vi "Test Performance.vi"() -> ()   [LabVIEW 2019]
uses:
  src/Typedefs/Interpolation Configuration--cluster.ctl
  <vilib>/Analysis/baseanly.llb/Mean.vi
  <vilib>/Analysis/baseanly.llb/Mean (DBL).vi
  src/xy_utilities.lvlib
panel:
  in  "Configure":T1={"X Low"=0.0, "X High"=1.0, "X Step"=0.1, "Fake Point"=0.0} {"Fake Point" format="%#_6p"; "X Step" format="%#_6p"; "X High" format="%#_6p"; "X Low" format="%#_6p"}
  out "XY Data 3":cluster{"X-array":dbl[], dbl[]}[](graph)
  out "Intensity Graph 2":dbl[][](graph)
  out "Intensity Graph":dbl[][](graph)
  out "execution time (s)":dbl
  out "XY Data 2":cluster{"X-array":dbl[], "Y-array":dbl[]}(graph)
  out "XY Data":cluster{"X-array":dbl[], "Y-array":dbl[]}(graph)
  # "0: 21\"\n5: 0.09\""
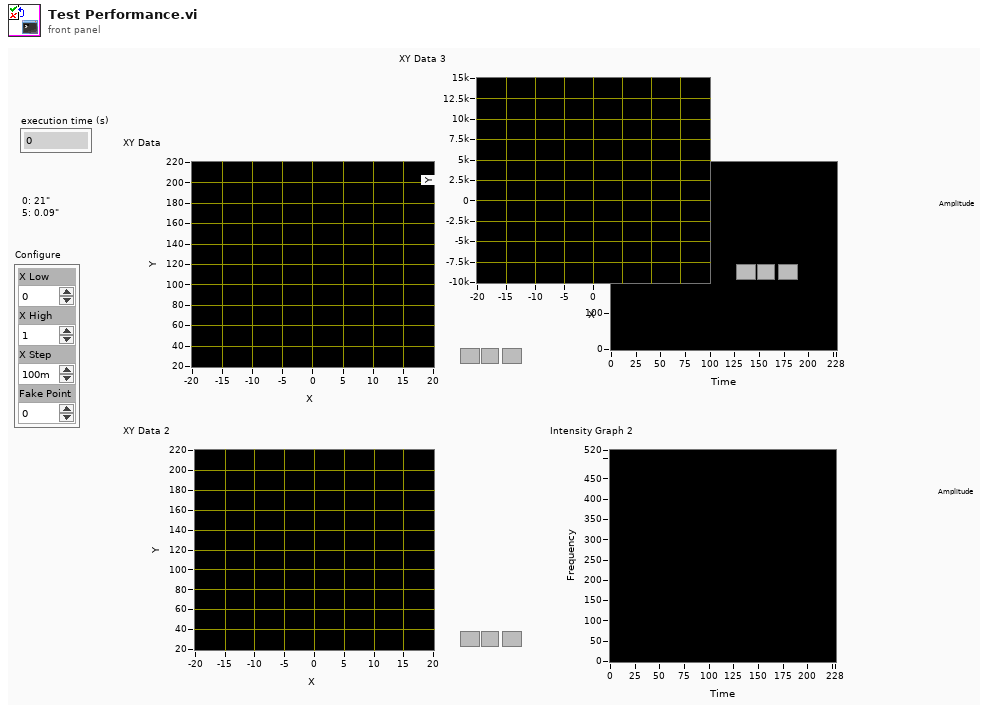
[diagram p1: front panel]
types:
  T1 = typedef "xy_utilities.lvlib/Interpolation Configuration--cluster.ctl" = cluster{"X Low":dbl, "X High":dbl, "X Step":dbl, "Fake Point":dbl}
  T2 = enum16{"thermal waveguide", "superlattice waveguide", "decay in atmosphere"}
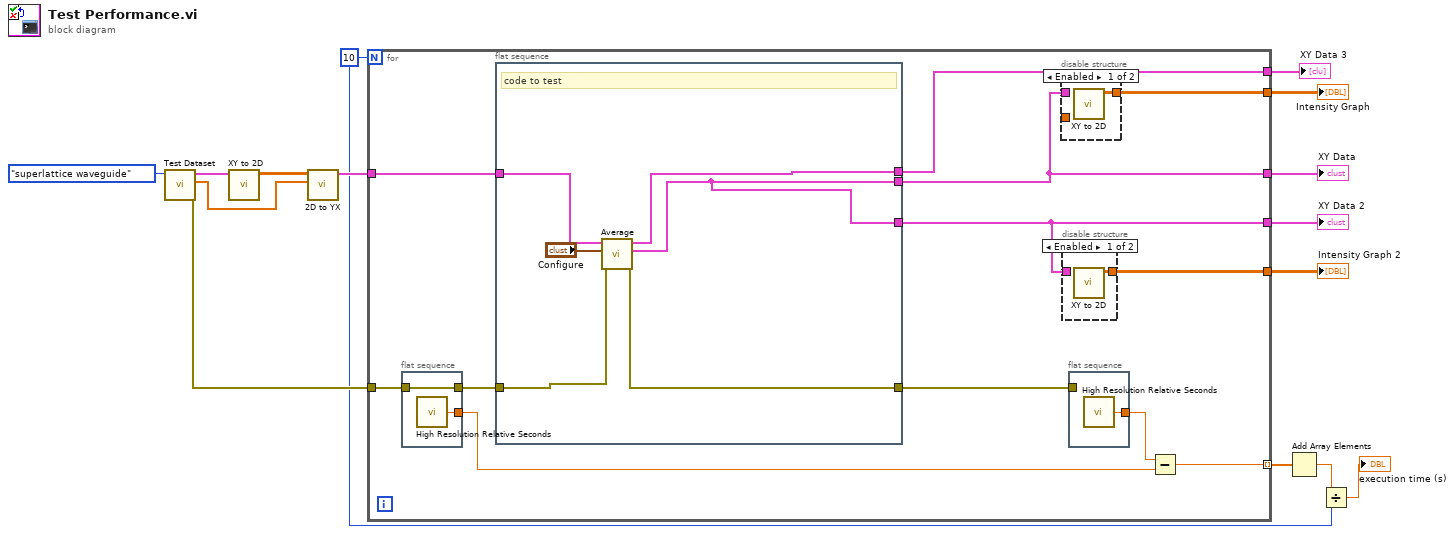
[diagram p0: block diagram]
diagram:
  w3 = 10
  n1 = call "Test Dataset.vi"("Enum"=T2."superlattice waveguide") -> ("error out"=w15:errorcluster, "Parameters out"=w7:dbl[], "XY-data out"=w8:cluster{"X-array":dbl[], "Y-array":dbl[]}[])  [unwired: 8 in]
  n2 = call "XY to 2D.vi"("XY-data"=w8) -> ("2D Z Array"=w6:dbl[][])  [unwired: 7 in, 3 out]
  n3 = call "2D to YX.vi"("Y Array"=w7, "2D Z Array"=w6) -> ("XY-data out"=w5:cluster{"X-array":dbl[], "Y-array":dbl[]}[])  [unwired: 8 in, 1 out]
  n4 = for {
    N: w3 -> [_]
    tunnel: w15 -> [w27]
    tunnel: w5 -> [w24]
    tunnel: [w17] -> w14
    tunnel: [w23] -> w13
    tunnel: [w22] -> w12
    tunnel: [w18] -> w11
    tunnel: [w19] -> w9 mode=indexing
    tunnel: [w16] -> w4
    n5 = flat-sequence {
      tunnel: [w39] -> w21
      tunnel: w27 -> [w39]
      tunnel: [w38] -> w25
      frame #0 {
        n6 = call <vilib>:"High Resolution Relative Seconds.vi"() -> ("relative seconds"=w38:dbl)
      }
    }
    n7 = flat-sequence {
      tunnel: w24 -> [w36]
      tunnel: [w34] -> w17
      tunnel: w21 -> [w33]
      tunnel: [w32] -> w20
      tunnel: [w34] -> w18
      tunnel: [w35] -> w16
      frame #0 {
        # "code to test"
        n8 = call "Average.vi"("error in (no error)"=w33, "Configure"="Configure", "XY-data"=w36) -> ("error out"=w32:errorcluster, "Averaged XY-data out"=w34:cluster{"X-array":dbl[], "Y-array":dbl[]}, "XY-data out"=w35:cluster{"X-array":dbl[], "Y-array":dbl[]}[])  [unwired: 6 in]
      }
    }
    n9 = disable-structure shown="Enabled" {
      disable-tunnel: [w29 w30] -> w22
      disable-tunnel: w18 -> [_ _]
      disable-tunnel: _ -> [_ w30]
      frame Enabled {
        n10 = call "XY to 2D.vi"() -> ("2D Z Array"=w29:dbl[][])  [unwired: 8 in, 3 out]
      }
      frame Disabled {
      }
    }
    n11 = disable-structure shown="Enabled" {
      disable-tunnel: [w28 _] -> w23
      disable-tunnel: w17 -> [_ _]
      frame Enabled {
        n12 = call "XY to 2D.vi"() -> ("2D Z Array"=w28:dbl[][])  [unwired: 8 in, 3 out]
      }
      frame Disabled {
      }
    }
    n13 = flat-sequence {
      tunnel: [w37] -> w26
      tunnel: w20 -> [_]
      frame #0 {
        n14 = call <vilib>:"High Resolution Relative Seconds.vi"() -> ("relative seconds"=w37:dbl)
      }
    }
    n15 = Subtract(x=w26, y=w25) -> (x-y=w19:dbl)
  }
  "XY Data" <- w11
  "XY Data 2" <- w14
  "Intensity Graph" <- w12
  "Intensity Graph 2" <- w13
  "XY Data 3" <- w4
  n16 = Add Array Elements(numeric array=w9) -> (sum=w2:dbl)
  n17 = Divide(x=w2, y=w3) -> (x/y=→"execution time (s)":dbl)
